vi "Request Compatible Hardware.vi"(8 "error in (no error)":errorcluster, 11 "Fcn UI in":refnum<class "Controller UI.lvclass">) -> (0 "error out":errorcluster, 3 "Fcn UI out":refnum<class "Controller UI.lvclass">)   [LabVIEW 2016, in "Controller UI.lvlib" / "Controller UI.lvclass"]
uses:
  <userlib>/Common Components/Controller UI/Controller UI.lvclass
  C:/Program Files (x86)/National Instruments/LabVIEW 2016/vi.lib/ActorFramework/Actor/Actor.lvclass
  <userlib>/Common Components/Controller UI/Controller UI.lvclass/Controller UI.ctl
  <vilib>/ActorFramework/Actor/Actor.lvclass/Actor.ctl
  <userlib>/Common Components/Controller/Messages/Find Compatible Hardware for Function Msg/Find Compatible Hardware for Function Msg.lvclass/Find Compatible Hardware for Function Msg.ctl
  <vilib>/ActorFramework/Message Enqueuer/Message Enqueuer.lvclass/Message Enqueuer.ctl
  <userlib>/Common Components/Controller UI/Accessors/Read Function.vi
  <vilib>/ActorFramework/Message Enqueuer/Enqueue.vi
  <userlib>/Common Components/Controller/Messages/Find Compatible Hardware for Function Msg/Find Compatible Hardware for Function Msg.lvclass
  C:/Program Files (x86)/National Instruments/LabVIEW 2016/vi.lib/ActorFramework/Message/Message.lvclass
  <vilib>/ActorFramework/Message Priority Queue/Priority Enqueue.vi
  <vilib>/ActorFramework/Actor/Actor.lvclass
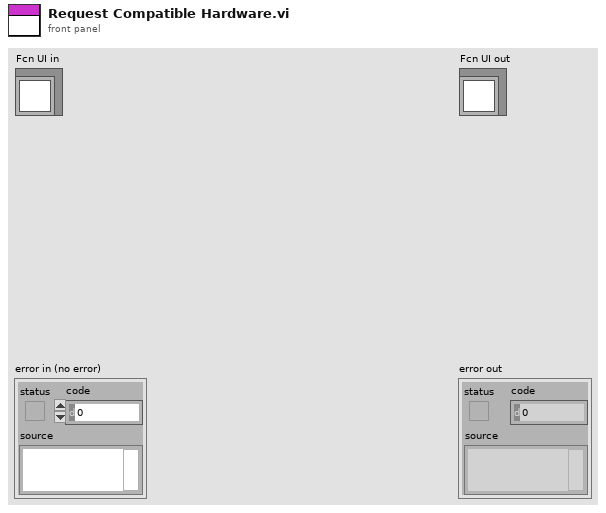
[diagram p1: front panel]
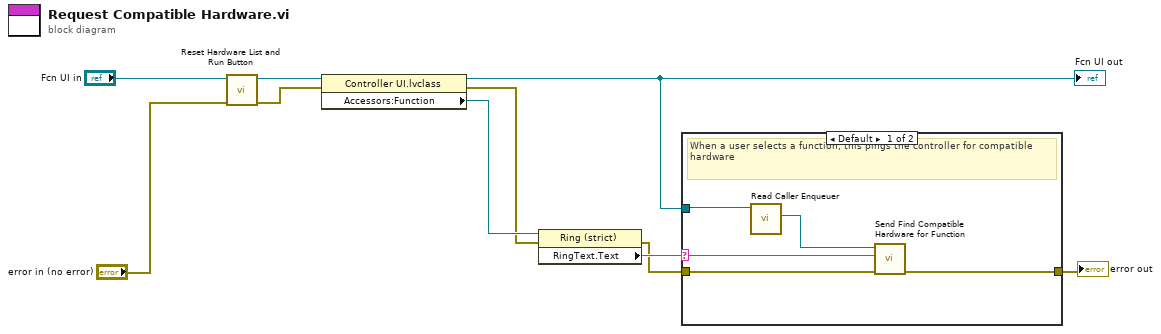
[diagram p0: block diagram]
diagram:
  n1 = call <userlib>:"Reset Hardware List and Run Button.vi"("error in (no error)"="error in (no error)", "Function UI in"="Fcn UI in") -> ("error out"=w2:errorcluster, "Function UI out"=w8:refnum<class "Controller UI.lvclass">)  [unwired: 8 in]
  n2 = property class="Controller UI.lvclass"(reference=w8, error in=w2) -> (reference out=w7:refnum<class "Controller UI.lvclass">, error out=w4:errorcluster, "Accessors:Function"=w6:refnum<vi>)
  "Fcn UI out" <- w7
  n3 = property class="Ring (strict)"(reference=w6, error in=w4) -> (error out=w3:errorcluster, "RingText.Text"=w10:string)  [unwired: 1 out]
  n4 = case shown="Default" w10 {
    selector: w10 -> [w13 _]
    tunnel: w7 -> [w15 _]
    tunnel: w3 -> [w12 w16]
    tunnel: [w11 w16] -> w1
    frame Default {
      # "When a user selects a function, this pings the controller for compatible hardware"
      n5 = call <vilib>:"Read Caller Enqueuer.vi"("Actor"=w15) -> ("Caller Enqueuer"=w14:refnum<class "Message Enqueuer.lvclass">)  [unwired: 10 in]
      n6 = call <userlib>:"Send Find Compatible Hardware for Function.vi"("error in (no error)"=w12, "Function Name"=w13, "Message Enqueuer"=w14) -> ("error out"=w11:errorcluster)  [unwired: 7 in, 1 out]
    }
    frame "Select One:" {
    }
  }
  "error out" <- w1
